vi "ziClose.vi"(3 "Error In":errorcluster, 5 "Handle In":T1 {"Handle" format="0x%08x"; "Conn" format="0x%08x"}) -> (0 "Error Out":errorcluster, 2 "Handle Out":T1 {"Handle" format="0x%08x"; "Conn" format="0x%08x"})   [LabVIEW 2015, in "Zurich Instruments LabOne.lvlib"]
doc: "Disconnects from a ziServer and frees resources. Use this vi to terminate a connection."
uses:
  <instrlib>/Zurich Instruments LabOne/Zurich Instruments LabOne.lvlib
  <instrlib>/Zurich Instruments LabOne/Public/ziTypeHandle.ctl
  <instrlib>/Zurich Instruments LabOne/Private/ziLV64.dll
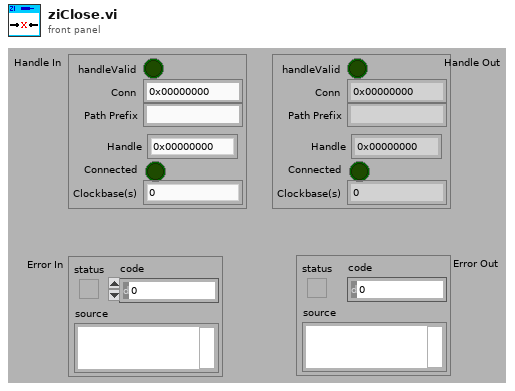
[diagram p1: front panel]
types:
  T1 = typedef "Zurich Instruments LabOne.lvlib/ziTypeHandle.ctl" = cluster{"handleValid":bool, "Conn":u64, "Path Prefix":string, "Handle":u64, "Connected":bool, "Clockbase(s)":dbl}
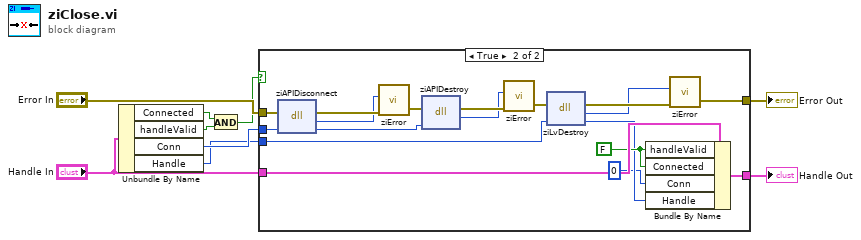
[diagram p0: block diagram]
diagram:
  n1 = Unbundle By Name("Handle In") -> ("Connected"=w2:bool, "handleValid"=w1:bool, "Conn"=w5:u64, "Handle"=w4:u64)
  n2 = And(x=w2, y=w1) -> (x .and. y?=w3:bool)
  n3 = case shown="True" w3 {
    tunnel: w5 -> [_ w29]
    tunnel: "Handle In" -> [w11 w28]
    tunnel: [w11 w27] -> w8
    tunnel: "Error In" -> [w10 w21]
    tunnel: [w10 w19] -> w7
    tunnel: w4 -> [_ w24]
    frame False {
    }
    frame True {
      w25 = FALSE ("handleOK")
      n4 = dll-call lib="C:/Program Files/National Instruments/LabVIEW 2015/instr.lib/Zurich Instruments LabOne/Private/ziLV*.*" fn="ziAPIDisconnect"(error in=w21, "Connection"=w29) -> (error out=w15:errorcluster, "return type"=w12:u32, "Connection"=w26:u64)  [unwired: 2 in, 1 out]
      n5 = call <instrlib>:"ziError.vi"("ziErrorCode"=w12, "Error In"=w15) -> ("Error Out"=w16:errorcluster)  [unwired: 4 in]
      n6 = dll-call lib="C:/Program Files/National Instruments/LabVIEW 2015/instr.lib/Zurich Instruments LabOne/Private/ziLV*.*" fn="ziAPIDestroy"(error in=w16, "Connection"=w26) -> (error out=w17:errorcluster, "return type"=w13:u32)  [unwired: 3 in, 1 out]
      n7 = call <instrlib>:"ziError.vi"("ziErrorCode"=w13, "Error In"=w17) -> ("Error Out"=w18:errorcluster)  [unwired: 4 in]
      n8 = dll-call lib="C:/Program Files/National Instruments/LabVIEW 2015/instr.lib/Zurich Instruments LabOne/Private/ziLV*.*" fn="ziLvDestroy" label="ziLVDestroy"(error in=w18, "Handle"=w24) -> (error out=w20:errorcluster, "return type"=w14:u32, "Handle"=w23:u64)  [unwired: 2 in, 1 out]
      n9 = Bundle By Name(cluster=w28, "handleValid"=w25, "Connected"=w25, "Conn"=u64 0, "Handle"=w23) -> (w27:T1)
      n10 = call <instrlib>:"ziError.vi"("ziErrorCode"=w14, "Error In"=w20) -> ("Error Out"=w19:errorcluster)  [unwired: 4 in]
    }
  }
  "Handle Out" <- w8
  "Error Out" <- w7
